vi "07.3 Loops with hardware API.vi"() -> ()   [LabVIEW 2019]
uses:
  <vilib>/DAQmx/read.llb/DAQmx Read (Analog Wfm 1Chan NSamp).vi
  <vilib>/DAQmx/create/channels.llb/DAQmx Create Channel (AI-Voltage-Basic).vi
  <vilib>/DAQmx/configure/timing.llb/DAQmx Timing (Sample Clock).vi
  <vilib>/DAQmx/miscellaneous.llb/DAQmx Fill In Error Info.vi
  <resource>/objmgr/daqmx.rc
panel:
  in  "Sample rate (Hz)":dbl=1000.0
  out "Actual Sample Rate":dbl
  in  "Stop":bool
  out "Data":waveform(dbl)(graph)
  in  "samples per channel":i32
  in  "Max value":dbl
  in  "Min value":dbl
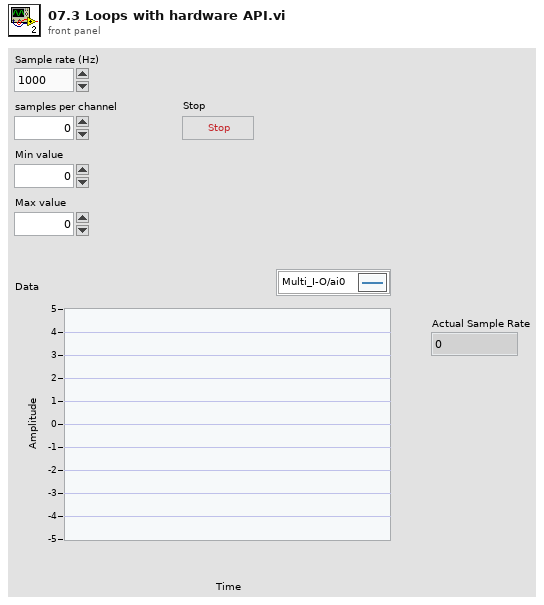
[diagram p1: front panel]
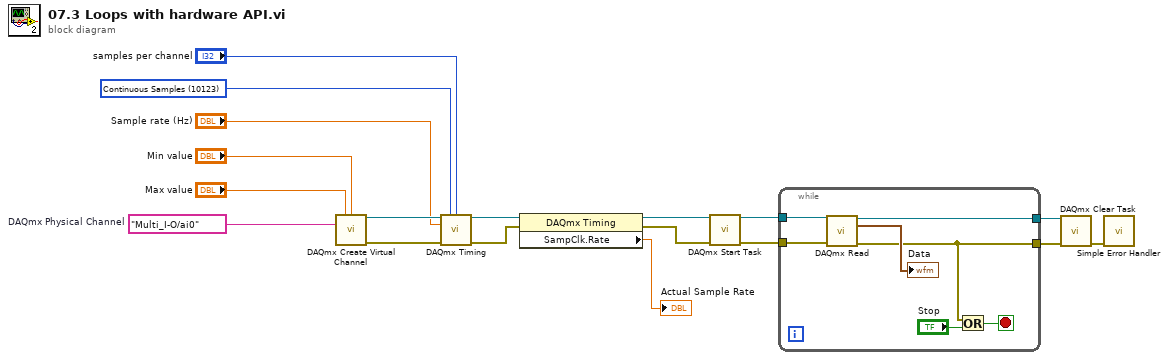
[diagram p0: block diagram]
diagram:
  w17 = 10123 items=["Finite Samples"=10178, "Continuous Samples"=10123, "Hardware Timed Single Point"=12522] ("sample mode")
  w18 = tag "Multi_I-O/ai0"  # DAQmx Physical Channel
  n1 = call-poly <vilib>:"DAQmx Create Virtual Channel.vi"("maximum value"="Max value", "minimum value"="Min value", "physical channels"=w18) -> ("task out"=w15:refnum<k21>, "error out"=w14:errorcluster)  [unwired: 11 in]
  n2 = call-poly <vilib>:"DAQmx Timing.vi"("task/channels in"=w15, "sample mode"=w17, "samples per channel"="samples per channel", "rate"="Sample rate (Hz)", "error in"=w14) -> ("task out"=w6:refnum<k21>, "error out"=w3:errorcluster)  [unwired: 9 in]
  n3 = property class="DAQmx Timing"(reference=w6, error in=w3) -> (reference out=w5:refnum<k21>, error out=w4:errorcluster, "SampClk.Rate"=→"Actual Sample Rate":dbl)
  n4 = call <vilib>:"DAQmx Start Task.vi"("task/channels in"=w5, "error in"=w4) -> ("task out"=w11:refnum<k21>, "error out"=w10:errorcluster)  [unwired: 12 in]
  n5 = while {
    tunnel: w11 -> [w24]
    tunnel: w10 -> [w25]
    tunnel: [w20] -> w9
    tunnel: [w19] -> w8
    stop <- w21 stop-if-true
    n6 = call-poly <vilib>:"DAQmx Read.vi"("task/channels in"=w24, "error in"=w25) -> ("task out"=w19:refnum<k21>, "data"=→"Data":waveform(dbl), "error out"=w20:errorcluster)  [unwired: 11 in]
    n7 = Or(x=w20, y="Stop") -> (x .or. y?=w21:bool)
  }
  n8 = call <vilib>:"DAQmx Clear Task.vi"("task in"=w8, "error in"=w9) -> ("error out"=w7:errorcluster)  [unwired: 13 in]
  n9 = call <vilib>:"Simple Error Handler.vi"("error in (no error)"=w7) -> ()  [unwired: 4 in, 5 out]
